vi "UI Controller.vi"(7 "Name (\"\" to Use UUID)":string="UI Controller") -> ()   [LabVIEW 2020]
uses:
  7d187395-4702-4f48-a3f4-ebc70eba639a.vi
  <userlib>/_NEVSTOP/Communicable State Machine(CSM)/AdvanceAPI/CSM - Revert Arguments-Safe String.vi
  <userlib>/_NEVSTOP/Communicable State Machine(CSM)/_Shared/Trim Single-line Text.vi
  <userlib>/_NEVSTOP/Communicable State Machine(CSM)/AdvanceAPI/CSM - Make String Arguments Safe.vi
  <userlib>/_NEVSTOP/Communicable State Machine(CSM)/AdvanceAPI/CSM - Break Down Multiple States String.vi
  <userlib>/_NEVSTOP/Communicable State Machine(CSM)/AdvanceAPI/CSM - Keywords.vi
  <userlib>/_NEVSTOP/Communicable State Machine(CSM)/addons/API-String-Arugments-Support/_Support/Data To API String Arguments.vi
  <userlib>/_NEVSTOP/Communicable State Machine(CSM)/Communicable State Machine.lvlib
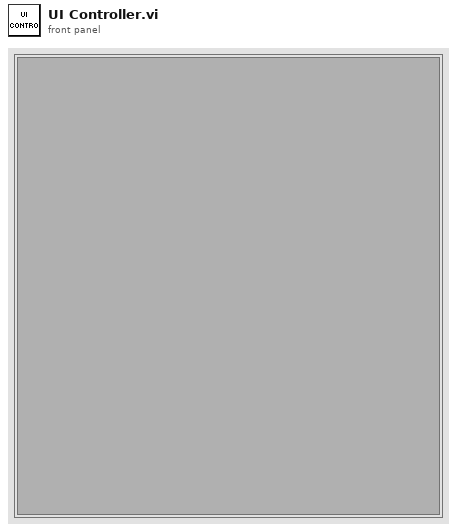
[diagram p1: front panel]
types:
  T1 = cluster{"Ref":cluster{"Name (\"\" to Use UUID)":refnum<vi>}, "Val":cluster{string}}
  T2 = cluster{"Current VI Reference":refnum<vi>, "Close Panel on Exit?":bool}
  T3 = cluster{"Core":cluster{"Current VI Reference":refnum<vi>, "Close Panel on Exit?":bool}, "1":cluster{"Ref":cluster{"Name (\"\" to Use UUID)":refnum<vi>}, "Val":cluster{string}}}
  T4 = enum32{"Invalid", "Standard", "Closed", "Hidden", "Minimized", "Maximized"}
  T5 = enum32{"invalid app kind", "Development System", "Run Time System", "Student Edition", "Embedded LabVIEW", "Evaluation", "Custom"}
  T6 = typedef "Communicable State Machine.lvlib/_CSM_Response Source Message.ctl" = cluster{"‘State":string, "’Arguments":string, "’Error":errorcluster}
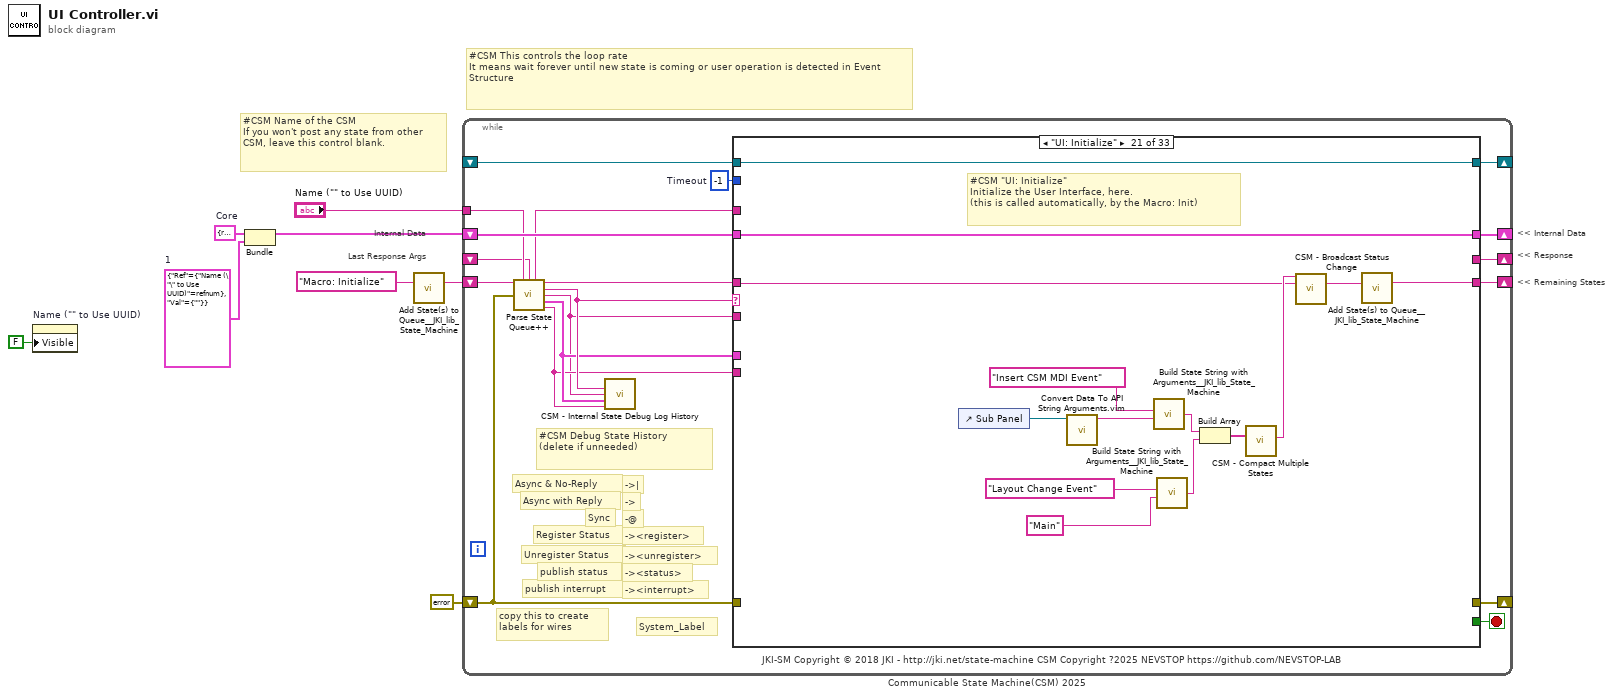
[diagram p0: block diagram]
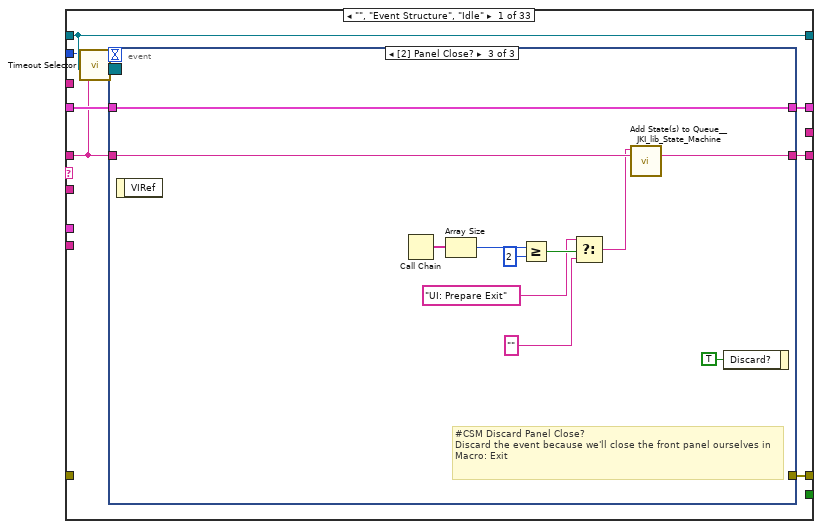
[diagram p2: hidden frame]
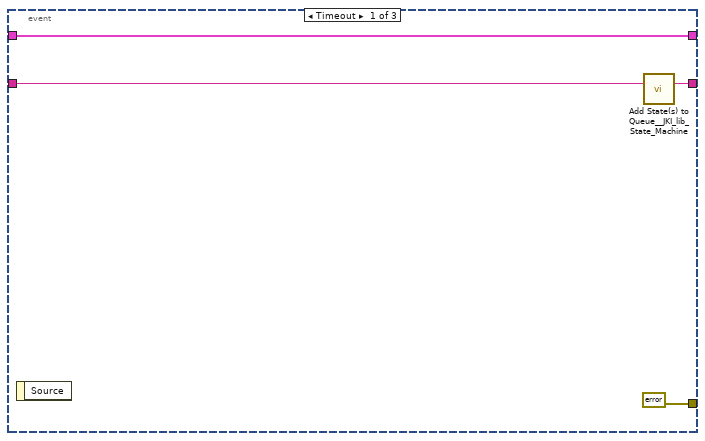
[diagram p3: hidden frame]
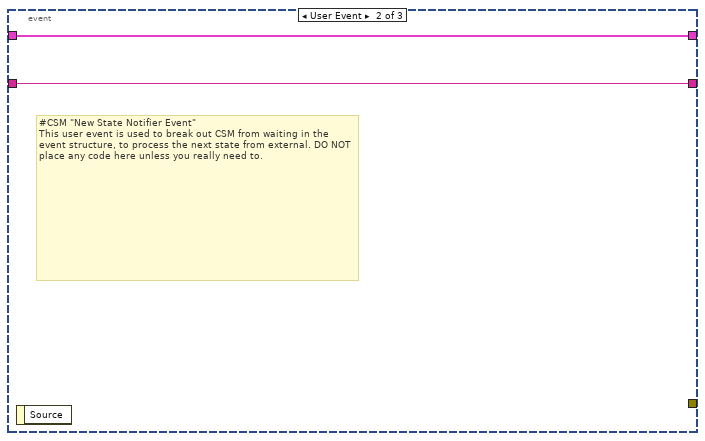
[diagram p4: hidden frame]
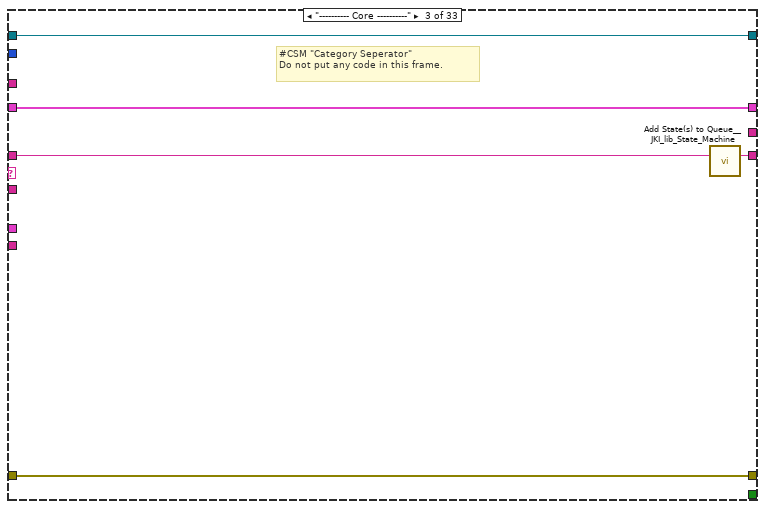
[diagram p6: hidden frame]
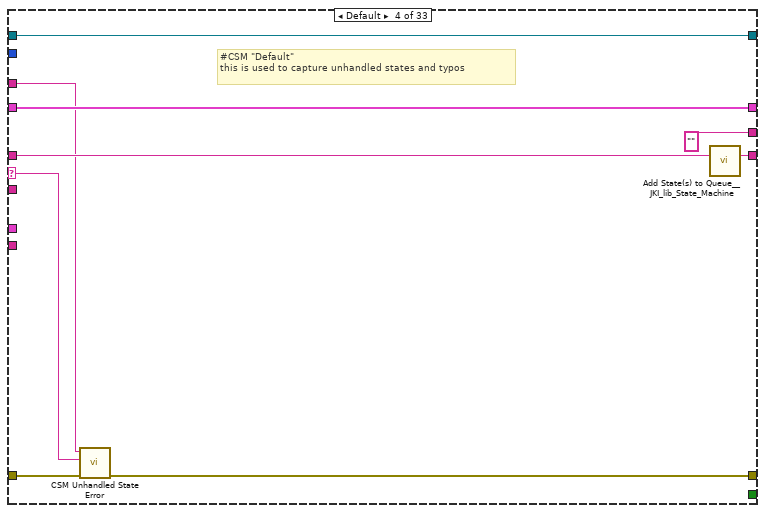
[diagram p7: hidden frame]
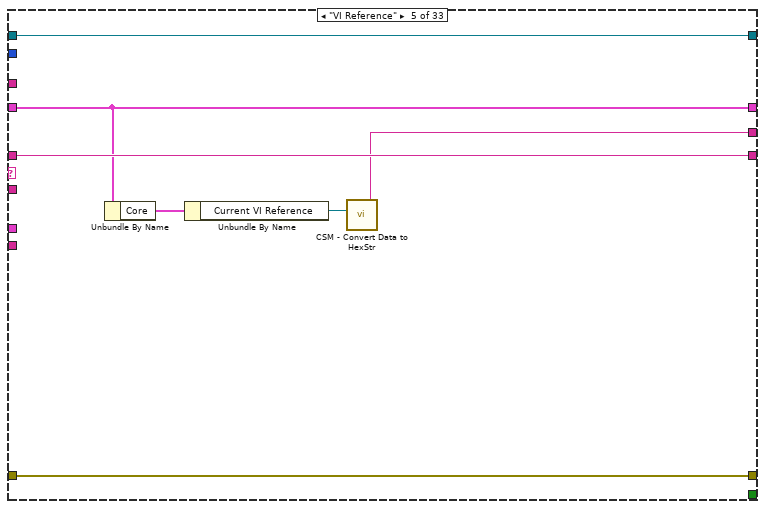
[diagram p8: hidden frame]
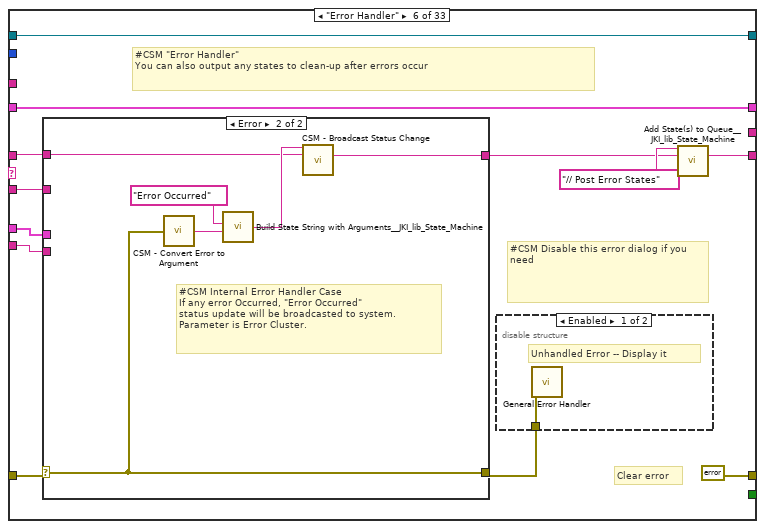
[diagram p9: hidden frame]
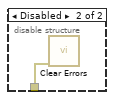
[diagram p10: hidden frame]
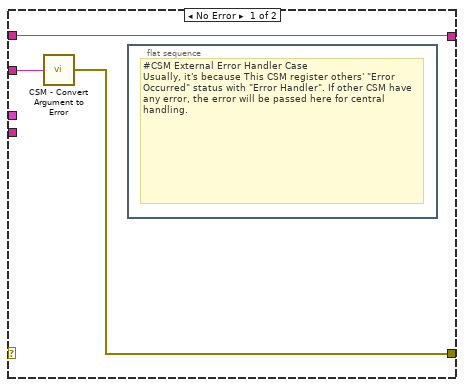
[diagram p11: hidden frame]
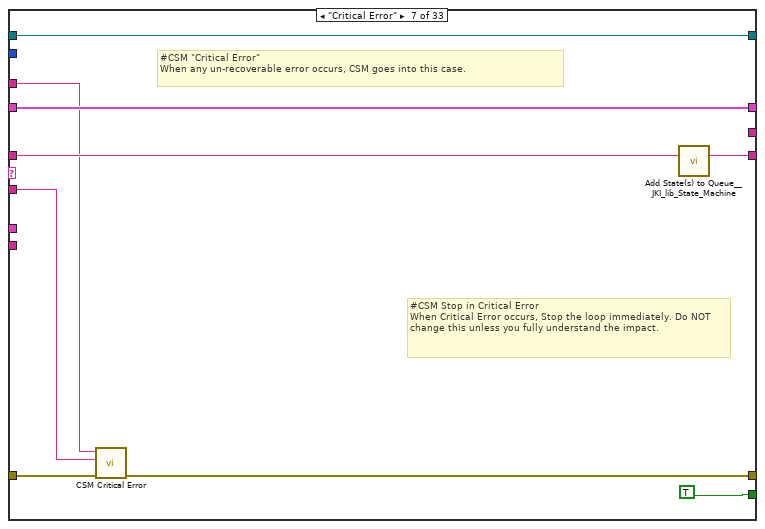
[diagram p12: hidden frame]
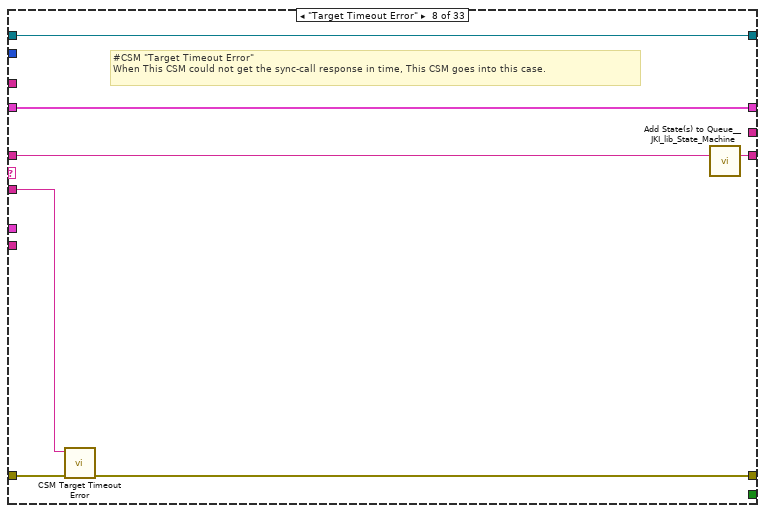
[diagram p13: hidden frame]
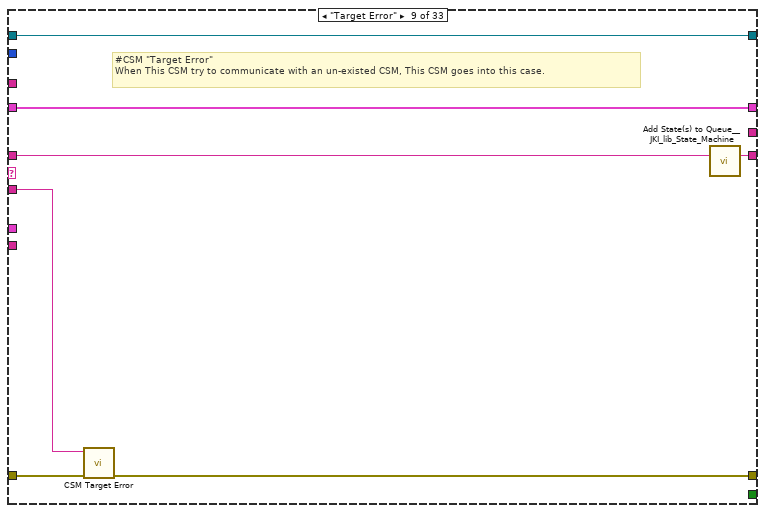
[diagram p14: hidden frame]
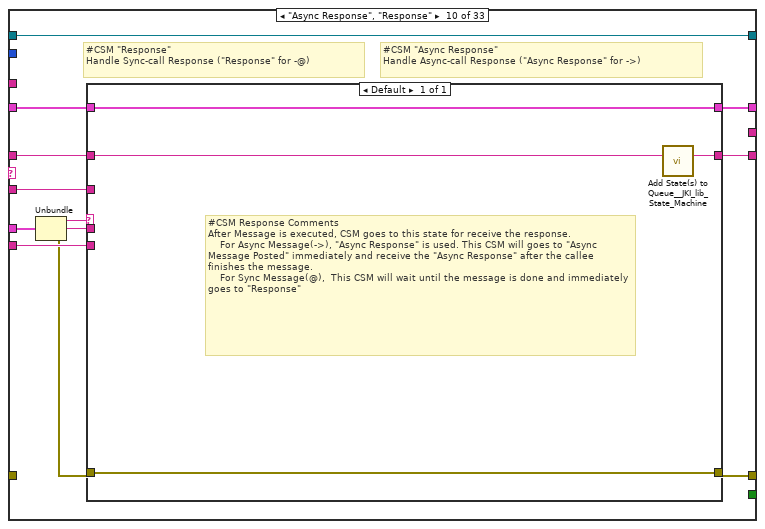
[diagram p15: hidden frame]
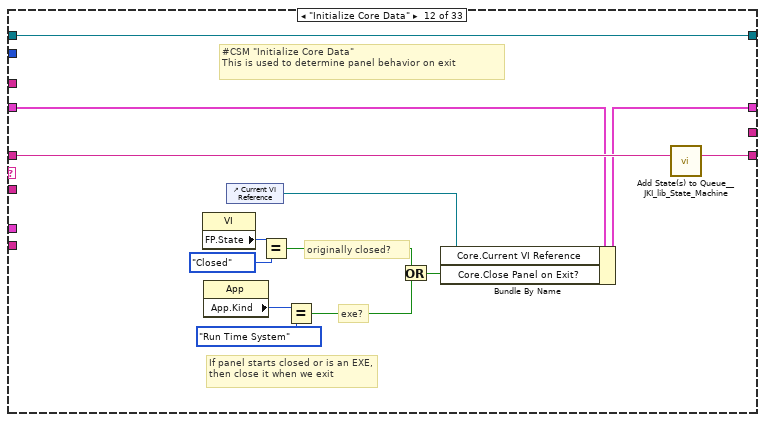
[diagram p17: hidden frame]
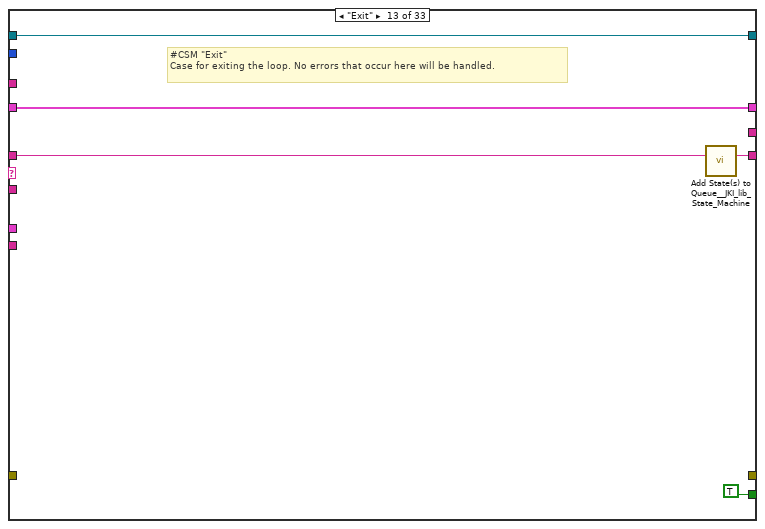
[diagram p18: hidden frame]
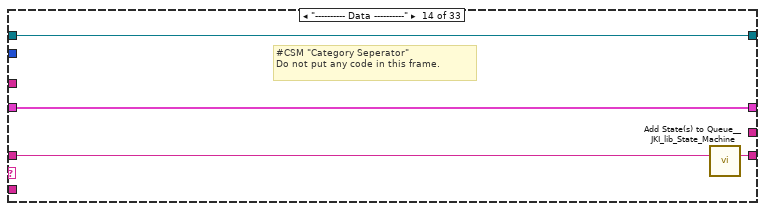
[diagram p19: hidden frame]
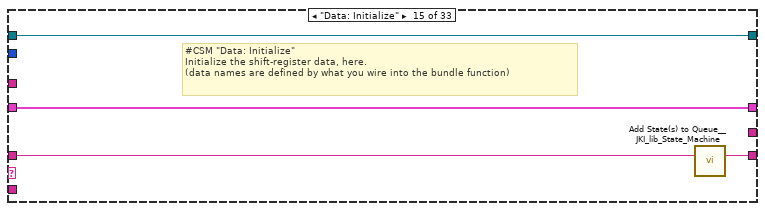
[diagram p20: hidden frame]
diagram:
  w7 = T1 {"Ref"={"Name (\"\" to Use UUID)"=refnum}, "Val"={""}}  # 1
  w6 = T2 {"Current VI Reference"=refnum, "Close Panel on Exit?"=FALSE}  # Core
  # "Last Response Args"
  # "Internal Data"
  # "<< Internal Data"
  # "<< Response"
  # "<< Remaining States"
  # "#CSM Name of the CSM\nIf you won't post any state from other CSM, leave this control blank."
  # "#CSM This controls the loop rate\nIt means wait forever until new state is coming or user operation is detected in Event Structure"
  n1 = property on="Name (\"\" to Use UUID)" class="Str"("Visible"=FALSE) -> ()  [unwired: 2 in, 2 out]
  n2 = Bundle("Core"=w6, "1"=w7) -> (w8:T3)  [unwired: 1 in]
  n3 = call <vilib>:"Add State(s) to Queue__JKI_lib_State_Machine.vi"("State(s) in (\"\")"="Macro: Initialize" ("Init State(\"Macro: Initialize\")")) -> ("States Out"=w2:string)  [unwired: 14 in]
  n4 = while "Communicable State Machine(CSM) 2025" {
    shift-right: [w22] -> _
    shift-left: w8 -> [w21]
    shift-right: [w25] -> _
    shift-left: errorcluster {"status"=FALSE, "code"=0, "source"=""} ("error out") -> [w19]
    shift-right: [w24] -> _
    shift-left: w2 -> [w26]
    tunnel: "Name (\"\" to Use UUID)" -> [w15]
    shift-right: [w18] -> _
    shift-left: _ -> [w10]
    shift-right: [w17] -> _
    shift-left: _ -> [w16]
    stop <- w23 stop-if-true
    w20 = -1  # Timeout
    # "#CSM Debug State History\n(delete if unneeded)"
    # "-><interrupt>"
    # "-><status>"
    # "-><unregister>"
    # "-><register>"
    # "-@"
    # "->"
    # "->|"
    # "publish interrupt"
    # "publish status"
    # "Unregister Status"
    # "Register Status"
    # "Sync"
    # "Async with Reply"
    # "Async & No-Reply"
    # "copy this to create labels for wires"
    # "System_Label"
    # "JKI-SM Copyright © 2018 JKI - http://jki.net/state-machine CSM Copyright ?2025 NEVSTOP https://github.com/NEVSTOP-LAB"
    n5 = call <userlib>:"Parse State Queue++.vi"("State Queue"=w26, "Name (\"\" to Use UUID)"=w15, "Response Arguments"=w10, "Previous Error"=w19) -> ("Name Used"=w11:string, "Remaining States"=w27:string, "Current State"=w14:string, "Arguments"=w9:string, "Additional Information"=w13:T6, "Source CSM"=w12:string)  [unwired: 6 in]
    n6 = call <userlib>:"CSM - Internal State Debug Log History.vi"("State"=w14, "Arguments (\"\")"=w9, ">> Response Source Message >>"=w13, "Source (\"\")"=w12) -> ()  [unwired: 11 in, 1 out]
    n7 = case shown="\"UI: Initialize\"" w14 {
      selector: w14 -> [_ _ _ w63 _ _ _ _ _ _ _ _ _ _ _ _ _ _ _ _ _ _ _ _ _ _ _ _ _ _ _ _ _]
      tunnel: w27 -> [w28 w55 w60 w69 w75 w81 w107 w115 w122 w132 w141 w154 w159 w163 w167 w173 w177 w184 w188 w192 w193 w208 w228 w239 w303 w304 w319 w322 w325 w330 w334 w338 w342]
      tunnel: w9 -> [_ _ _ _ _ w79 w103 w110 w118 w126 _ _ _ _ _ _ _ _ _ _ _ _ w224 w234 _ _ _ _ _ _ _ _ _]
      tunnel: w21 -> [w34 w54 w57 w67 w74 w87 w108 w113 w120 w130 w140 w148 w157 w161 w164 w169 w175 w183 w187 w190 w205 w215 w226 w236 w301 w307 w317 w321 w327 w329 w332 w336 w340]
      tunnel: [w33 _ w58 w61 w76 errorcluster {"status"=FALSE, "code"=0, "source"=""} ("error out") w100 w109 w116 w129 _ _ _ _ _ w170 _ w178 w186 _ _ _ w225 w237 _ _ _ _ _ _ _ _ _] -> w25
      tunnel: w19 -> [_ _ w58 w62 w76 w85 w101 w111 w117 _ _ _ _ _ _ _ _ _ _ _ _ _ _ _ _ _ _ _ _ _ _ _ _]
      tunnel: [w35 w55 w59 w68 w75 w83 w106 w114 w121 w133 w141 w153 w158 w162 w166 w172 w176 w184 w188 w191 w206 w209 w227 w238 w302 w308 w318 w322 w324 w330 w333 w337 w341] -> w24
      tunnel: [_ _ _ _ _ _ TRUE _ _ _ _ _ TRUE _ _ _ _ _ _ _ _ _ _ _ _ _ _ _ _ _ _ _ _] -> w23
      tunnel: [w32 w54 w57 w67 w74 w87 w108 w113 w120 w131 w140 w152 w157 w161 w164 w169 w175 w183 w187 w190 w205 w215 w226 w236 w301 w307 w317 w321 w327 w329 w332 w336 w340] -> w22
      tunnel: w20 -> [w30 _ _ _ _ _ _ _ _ _ _ _ _ _ _ _ _ _ _ _ _ _ _ _ _ _ _ _ _ _ _ _ _]
      tunnel: w12 -> [_ _ _ _ _ w78 _ _ _ w127 _ _ _ _ _ _ _ _ _ _ _ _ _ _ _ _ _ _ _ _ _ _ _]
      tunnel: w13 -> [_ _ _ _ _ w77 _ _ _ w128 _ _ _ _ _ _ _ _ _ _ _ _ _ _ _ _ _ _ _ _ _ _ _]
      tunnel: [_ _ _ "" w70 _ _ _ _ _ _ _ _ _ _ _ _ _ _ _ _ _ _ _ _ _ _ _ _ _ _ _ _] -> w18
      tunnel: [w31 w53 w56 w65 w73 w86 w104 w112 w119 w134 w139 w142 w155 w160 w165 w168 w174 w182 w185 w189 w204 w219 w223 w233 w300 w305 w311 w320 w326 w328 w331 w335 w339] -> w17
      tunnel: w16 -> [w31 w53 w56 w65 w73 w86 w104 w112 w119 w134 w139 w142 w155 w160 w165 w168 w174 _ w185 w189 w204 w219 w223 w233 w300 w305 w311 w320 w326 w328 w331 w335 w339]
      tunnel: w11 -> [_ _ _ w64 _ _ w102 _ _ _ _ _ _ _ _ _ _ w181 _ _ _ _ _ _ _ _ _ _ _ _ _ _ _]
      frame "", "Event Structure", "Idle" {
        n8 = call <userlib>:"Timeout Selector.vi"("Remaining States"=w28, "Timeout Expected"=w30) -> ("Timeout"=w29:i32)  [unwired: 5 in]
        n9 = event shown="[2] Panel Close?" {
          selector: w31 -> [_ _ _]
          dyn-events: _ -> [_ _ _]
          timeout: w29 -> [_ _ _]
          tunnel: w28 -> [w39 w40 w52]
          tunnel: [w38 w40 w51] -> w35
          tunnel: w34 -> [w37 w41 w50]
          tunnel: [errorcluster {"status"=FALSE, "code"=0, "source"=""} ("error out") _ _] -> w33
          tunnel: [w37 w41 w50] -> w32
          event Timeout {
            n10 = event-data() -> ()  [unwired: 1 in, 1 out]
            n11 = call <vilib>:"Add State(s) to Queue__JKI_lib_State_Machine.vi"("State(s) in (\"\")"=w39) -> ("States Out"=w38:string)  [unwired: 14 in]
          }
          event User Event {
            # "#CSM \"New State Notifier Event\"\nThis user event is used to break out CSM from waiting in the event structure, to process the next state from external. DO NOT place any code here unless you really need to."
            n12 = event-data() -> ()  [unwired: 1 in, 1 out]
          }
          event Panel Close? {
            # "#CSM Discard Panel Close?\nDiscard the event because we'll close the front panel ourselves in Macro: Exit"
            n13 = event-data() -> ()  [unwired: 1 in, 1 out]
            n14 = Call Chain() -> (call chain=w44:string[])
            n15 = Array Size(array=w44) -> (size(s)=w48:i32)
            n16 = Greater Or Equal?(x=w48, y=2) -> (x >= y?=w46:bool)
            n17 = Select(t="UI: Prepare Exit", s=w46, f="" ("t")) -> (s? t:f=w42:string)
            n18 = call <vilib>:"Add State(s) to Queue__JKI_lib_State_Machine.vi"("State(s) in Front (\"\")"=w42, "State(s) in (\"\")"=w52) -> ("States Out"=w51:string)  [unwired: 13 in]
            n19 = event-data("Discard?"=TRUE) -> ()  [unwired: 1 in, 1 out]
          }
        }
      }
      frame "CSM Documentation" {
        # "#CSM State Syntax\n\n// Comment line, all text to the right of “//” will be ignored\n// Local Message Example\nDoSth: DoA >> Arguments\n\n// Sync Call Example\nAPI: xxxx >> Arguments -@ TargetModule\n\n// Async Call Example\nAPI: xxxx >> Arguments -> TargetModule\n\n// Async Call without Reply Example\nAPI: xxxx >> Arguments ->| TargetModule\n\n// Broadcast normal status:\nStatus >> StatusArguments  -><status>\n\n// Broadcast Interrupt status:\nInterrupt >> StatusArguments  -><interrupt>\n\n// Register Source Module's status to Handler Module\nStatus@Source Module >> Handler Module@Handler Module -><register>\n\n// Unegister Source Module's status\nStatus@Source Module >> Handler Module -><unregister>"
        # "#CSM README FIRST\n\nCommunicable State Machine(CSM) is a LabVIEW application framework that builds upon JKI State Machine(JKISM). It follows the pattern of JKISM and extends the keywords to describe message communication between modules, including concepts such as Sync-Message, Async-Message, Subscription/Unsubscription of status - essential elements for creating reusable code modules. For more information, please visit the CSM wiki: https://nevstop-lab.github.io/CSM-Wiki/\n\nFor instructions on JKI State Machine, visit: \n    http://jki.net/state-machine/\nFor information about CSM, visit: \n    https://github.com/NEVSTOP-LAB"
        # "#CSM \"Documentation\"\nCase for holding CSM Documenation"
      }
      frame "---------- Core ----------" {
        # "#CSM \"Category Seperator\"\nDo not put any code in this frame."
        n20 = call <vilib>:"Add State(s) to Queue__JKI_lib_State_Machine.vi"("State(s) in (\"\")"=w60) -> ("States Out"=w59:string)  [unwired: 14 in]
      }
      frame Default {
        # "#CSM \"Default\"\nthis is used to capture unhandled states and typos"
        n21 = call <userlib>:"CSM Unhandled State Error.vi"("error in (no error)"=w62, "Undefined State"=w63, "CSM Name"=w64) -> ("error out"=w61:errorcluster)  [unwired: 8 in]
        n22 = call <vilib>:"Add State(s) to Queue__JKI_lib_State_Machine.vi"("State(s) in (\"\")"=w69) -> ("States Out"=w68:string)  [unwired: 14 in]
      }
      frame "VI Reference" {
        n23 = Unbundle By Name(w74) -> ("Core"=w72:T2)
        n24 = Unbundle By Name(w72) -> ("Current VI Reference"=w71:refnum<vi>)
        n25 = call <userlib>:"CSM - Convert Data to HexStr.vi"("Variant"=w71) -> ("HEX String (0-9,A-F)"=w70:string)  [unwired: 8 in]
      }
      frame "Error Handler" {
        # "#CSM Disable this error dialog if you need"
        # "#CSM \"Error Handler\"\nYou can also output any states to clean-up after errors occur"
        # "Clear error"
        n26 = case shown="Error" w85 {
          selector: w85 -> [_ w94]
          tunnel: [w92 w96] -> w82
          tunnel: w81 -> [w92 w95]
          tunnel: [w91 w94] -> w80
          tunnel: w79 -> [w93 _]
          tunnel: w78 -> [_ _]
          tunnel: w77 -> [_ _]
          frame No Error {
            n27 = call <userlib>:"CSM - Convert Argument to Error.vi"("Argument"=w93) -> ("Error"=w91:errorcluster)  [unwired: 4 in]
            n28 = flat-sequence {
              frame #0 {
                # "#CSM External Error Handler Case\nUsually, it's because This CSM register others' \"Error Occurred\" status with \"Error Handler\". If other CSM have any error, the error will be passed here for central handling."
              }
            }
          }
          frame Error {
            # "#CSM Internal Error Handler Case \nIf any error Occurred, \"Error Occurred\" \nstatus update will be broadcasted to system.\nParameter is Error Cluster."
            n29 = call <userlib>:"CSM - Convert Error to Argument.vi"("Error"=w94) -> ("Argument"=w98:string)  [unwired: 4 in]
            n30 = call <vilib>:"Build State String with Arguments__JKI_lib_State_Machine.vi"("Arguments (\"\")"=w98, "State"="Error Occurred" ("Status with Arguments")) -> ("State with Arguments"=w97:string)  [unwired: 4 in]
            n31 = call <userlib>:"CSM - Broadcast Status Change.vi"("Status With Arguments"=w97, "State Queue"=w95) -> ("Remaining States"=w96:string)  [unwired: 13 in]
          }
        }
        n32 = disable-structure shown="Enabled" {
          disable-tunnel: w80 -> [w89 w90]
          frame Enabled {
            # "Unhandled Error -- Display it"
            n33 = call <vilib>:"General Error Handler.vi"("error in (no error)"=w89) -> ()  [unwired: 10 in, 5 out]
          }
          frame Disabled {
            n34 = call <vilib>:"Clear Errors.vi"("error in (no error)"=w90) -> ()  [unwired: 5 in, 2 out]
          }
        }
        n35 = call <vilib>:"Add State(s) to Queue__JKI_lib_State_Machine.vi"("State(s) in Front (\"\")"="// Post Error States", "State(s) in (\"\")"=w82) -> ("States Out"=w83:string)  [unwired: 13 in]
      }
      frame "Critical Error" {
        # "#CSM \"Critical Error\"\nWhen any un-recoverable error occurs, CSM goes into this case."
        # "#CSM Stop in Critical Error\nWhen Critical Error occurs, Stop the loop immediately. Do NOT change this unless you fully understand the impact."
        n36 = call <userlib>:"CSM Critical Error.vi"("error in (no error)"=w101, "Arugments (As Reason)"=w103, "CSM Name"=w102) -> ("error out"=w100:errorcluster)  [unwired: 8 in]
        n37 = call <vilib>:"Add State(s) to Queue__JKI_lib_State_Machine.vi"("State(s) in (\"\")"=w107) -> ("States Out"=w106:string)  [unwired: 14 in]
      }
      frame "Target Timeout Error" {
        # "#CSM \"Target Timeout Error\"\nWhen This CSM could not get the sync-call response in time, This CSM goes into this case."
        n38 = call <userlib>:"CSM Target Timeout Error.vi"("error in (no error)"=w111, "Arguments (As CSM Name)"=w110) -> ("error out"=w109:errorcluster)  [unwired: 9 in]
        n39 = call <vilib>:"Add State(s) to Queue__JKI_lib_State_Machine.vi"("State(s) in (\"\")"=w115) -> ("States Out"=w114:string)  [unwired: 14 in]
      }
      frame "Target Error" {
        # "#CSM \"Target Error\"\nWhen This CSM try to communicate with an un-existed CSM, This CSM goes into this case."
        n40 = call <userlib>:"CSM Target Error.vi"("error in (no error)"=w117, "Arguments (As CSM Name)"=w118) -> ("error out"=w116:errorcluster)  [unwired: 9 in]
        n41 = call <vilib>:"Add State(s) to Queue__JKI_lib_State_Machine.vi"("State(s) in (\"\")"=w122) -> ("States Out"=w121:string)  [unwired: 14 in]
      }
      frame "Async Response", "Response" {
        # "#CSM \"Async Response\"\nHandle Async-call Response (\"Async Response\" for ->)"
        # "#CSM \"Response\"\nHandle Sync-call Response (\"Response\" for -@)"
        n42 = Unbundle(w128) -> ("‘State"=w125:string, "’Arguments"=w124:string, "’Error"=w123:errorcluster)
        n43 = case shown="Default" w125 {
          tunnel: [w135] -> w133
          tunnel: w132 -> [w136]
          tunnel: [w138] -> w131
          tunnel: w130 -> [w138]
          tunnel: [w137] -> w129
          tunnel: w123 -> [w137]
          tunnel: w127 -> [_]
          tunnel: w126 -> [_]
          tunnel: w124 -> [_]
          frame Default {
            # "#CSM Response Comments\nAfter Message is executed, CSM goes to this state for receive the response.\n    For Async Message(->), \"Async Response\" is used. This CSM will goes to \"Async Message Posted\" immediately and receive the \"Async Response\" after the callee finishes the message.\n    For Sync Message(@),  This CSM will wait until the message is done and immediately goes to \"Response\""
            n44 = call <vilib>:"Add State(s) to Queue__JKI_lib_State_Machine.vi"("State(s) in (\"\")"=w136) -> ("States Out"=w135:string)  [unwired: 14 in]
          }
        }
      }
      frame "Async Message Posted" {
        # "#CSM \"Async Message Posted\"\nAfter Async Message is posted (-> or ->| ), CSM goes to this state for post-action.\nYou can use Argument - State to tell which Async Message is called."
      }
      frame "Initialize Core Data" {
        # "#CSM \"Initialize Core Data\"\nThis is used to determine panel behavior on exit"
        # "originally closed?"
        # "exe?"
        # "If panel starts closed or is an EXE, then close it when we exit"
        n45 = property class="VI"() -> ("FP.State"=w145:T4)  [unwired: 2 in, 2 out]
        n46 = property class="App"() -> ("App.Kind"=w151:T5)  [unwired: 2 in, 2 out]
        n47 = control-ref of="Current VI Reference"() -> (w146:refnum<vi>)
        n48 = Equal?(x=w145, y=T4."Closed" ("Front Panel Window:State")) -> (x = y?=w143:bool)
        n49 = Equal?(x=w151, y=T5."Run Time System" ("Application:Kind")) -> (x = y?=w149:bool)
        n50 = Or(x=w143, y=w149) -> (x .or. y?=w147:bool)
        n51 = Bundle By Name(cluster=w148, "Core.Current VI Reference"=w146, "Core.Close Panel on Exit?"=w147) -> (w152:T3)
        n52 = call <vilib>:"Add State(s) to Queue__JKI_lib_State_Machine.vi"("State(s) in (\"\")"=w154) -> ("States Out"=w153:string)  [unwired: 14 in]
      }
      frame "Exit" {
        # "#CSM \"Exit\"\nCase for exiting the loop. No errors that occur here will be handled."
        n53 = call <vilib>:"Add State(s) to Queue__JKI_lib_State_Machine.vi"("State(s) in (\"\")"=w159) -> ("States Out"=w158:string)  [unwired: 14 in]
      }
      frame "---------- Data ----------" {
        # "#CSM \"Category Seperator\"\nDo not put any code in this frame."
        n54 = call <vilib>:"Add State(s) to Queue__JKI_lib_State_Machine.vi"("State(s) in (\"\")"=w163) -> ("States Out"=w162:string)  [unwired: 14 in]
      }
      frame "Data: Initialize" {
        # "#CSM \"Data: Initialize\"\nInitialize the shift-register data, here.\n(data names are defined by what you wire into the bundle function)"
        n55 = call <vilib>:"Add State(s) to Queue__JKI_lib_State_Machine.vi"("State(s) in (\"\")"=w167) -> ("States Out"=w166:string)  [unwired: 14 in]
      }
      frame "Data: Cleanup" {
        # "#CSM \"Data: Cleanup\"\nCleanup any data and references, here.\n(this is called automatically, by the Macro: Exit)"
        n56 = Unbundle By Name(w169) -> ("Core.Current VI Reference"=w171:refnum<vi>)
        n57 = Close Reference(reference=w171) -> (error out=w170:errorcluster)  [unwired: 1 in]
        n58 = call <vilib>:"Add State(s) to Queue__JKI_lib_State_Machine.vi"("State(s) in (\"\")"=w173) -> ("States Out"=w172:string)  [unwired: 14 in]
      }
      frame "---------- Events ----------" {
        # "#CSM \"Category Seperator\"\nDo not put any code in this frame."
        n59 = call <vilib>:"Add State(s) to Queue__JKI_lib_State_Machine.vi"("State(s) in (\"\")"=w177) -> ("States Out"=w176:string)  [unwired: 14 in]
      }
      frame "Events: Register" {
        # "#CSM \"Events: Register\"\nRegister user event. New Message Event is registered to break CSM waiting in event structure by default."
        # "#CSM Register New Message Event\nRegister message event to break Waiting in Event structure."
        n60 = call <userlib>:"CSM - Get New State Notifier Event.vi"("Name (\"\" to Use UUID)"=w181) -> ("error out"=w179:errorcluster, "New State Notifier Event"=w180:refnum<user-event>)  [unwired: 9 in]
        n61 = register-events(error in=w179, w180) -> (reference out=w182:refnum<event-registration>, error out=w178:errorcluster)  [unwired: 1 in]
      }
      frame "Events: Unregister" {
        # "#CSM \"Events: Unregister\"\nUnregister user event."
        n62 = Unregister For Events(event registration refnum=w185) -> (error out=w186:errorcluster)  [unwired: 1 in]
      }
      frame "---------- UI ----------" {
        # "#CSM \"Category Seperator\"\nDo not put any code in this frame."
        n63 = call <vilib>:"Add State(s) to Queue__JKI_lib_State_Machine.vi"("State(s) in (\"\")"=w192) -> ("States Out"=w191:string)  [unwired: 14 in]
      }
      frame "UI: Initialize" {
        # "#CSM \"UI: Initialize\"\nInitialize the User Interface, here.\n(this is called automatically, by the Macro: Init)"
        n64 = control-ref of="Sub Panel"() -> (w202:refnum<vi>)
        n65 = call "Convert Data To API String Arguments.vim"("Data"=w202) -> ("API String"=w203:string)  [unwired: 7 in, 1 out]
        n66 = call <vilib>:"Build State String with Arguments__JKI_lib_State_Machine.vi"("Arguments (\"\")"=w203, "State"="Insert CSM MDI Event") -> ("State with Arguments"=w197:string)  [unwired: 4 in]
        n67 = call <vilib>:"Build State String with Arguments__JKI_lib_State_Machine.vi"("Arguments (\"\")"="Main" ("y"), "State"="Layout Change Event") -> ("State with Arguments"=w196:string)  [unwired: 4 in]
        n68 = Build Array(w197, w196) -> (w195:string[])
        n69 = call <userlib>:"CSM - Compact Multiple States.vi"("Multiple States"=w195) -> ("States"=w194:string)  [unwired: 9 in]
        n70 = call <userlib>:"CSM - Broadcast Status Change.vi"("Status With Arguments"=w194, "State Queue"=w193) -> ("Remaining States"=w200:string)  [unwired: 13 in]
        n71 = call <vilib>:"Add State(s) to Queue__JKI_lib_State_Machine.vi"("State(s) in (\"\")"=w200) -> ("States Out"=w206:string)  [unwired: 14 in]
      }
      frame "UI: Prepare Exit" {
        w212 = "Main" ("y")
        n72 = Unbundle By Name(w215) -> ("Core.Current VI Reference"=w214:refnum<vi>)
        n73 = property class="VI"(reference=w214) -> ("Front Panel.Title"=w218:string)  [unwired: 1 in, 2 out]
        n74 = Not Equal?(x=w218, y=w212) -> (x != y?=w211:bool)
        n75 = case shown="True" w211 {
          tunnel: [_ w221] -> w207
          tunnel: w212 -> [_ w220]
          frame False {
          }
          frame True {
            n76 = call <vilib>:"Build State String with Arguments__JKI_lib_State_Machine.vi"("Arguments (\"\")"=w220, "State"="Layout Change Event" ("Status With Arguments")) -> ("State with Arguments"=w221:string)  [unwired: 4 in]
          }
        }
        n77 = Select(t="", s=w211, f="Macro: Exit") -> (s? t:f=w213:string)
        n78 = call <vilib>:"Add State(s) to Queue__JKI_lib_State_Machine.vi"("State(s) in Front (\"\")"=w213, "State(s) in (\"\")"=w208) -> ("States Out"=w210:string)  [unwired: 13 in]
        n79 = call <userlib>:"CSM - Broadcast Status Change.vi"("Status With Arguments"=w207, "State Queue"=w210) -> ("Remaining States"=w209:string)  [unwired: 13 in]
      }
      frame "UI: Cursor Set" {
        # "Argument"
        # "#CSM \"UI: Cursor Set\"\nSet and Unset Cursor Busy.\n(Usage: \"UI: Cursor Set >> Busy|Idle\")"
        n80 = disable-structure shown="TARGET_TYPE!=Windows" {
          disable-tunnel: [w230 _] -> w225
          disable-tunnel: w224 -> [w229 _]
          frame condition #0 (active) {
            n81 = case shown="\"Idle\", Default" w229 {
              tunnel: [w231 w232] -> w230
              frame "Idle", Default {
                n82 = call <vilib>:"Unset Busy.vi"() -> ("error out"=w231:errorcluster)  [unwired: 11 in]
              }
              frame "Busy" {
                n83 = call <vilib>:"Set Busy.vi"() -> ("error out"=w232:errorcluster)  [unwired: 10 in, 1 out]
              }
            }
          }
          frame condition #1 {
          }
        }
        n84 = call <vilib>:"Add State(s) to Queue__JKI_lib_State_Machine.vi"("State(s) in (\"\")"=w228) -> ("States Out"=w227:string)  [unwired: 14 in]
      }
      frame "UI: Front Panel State" {
        # "Argument"
        # "#CSM \"UI: Front Panel State\"\nSet Front Panel Open or Closed\n(Usage: \"UI: Front Panel State >> Open|Close\")"
        n85 = Unbundle By Name(w236) -> ("Core.Current VI Reference"=w235:refnum<vi>)
        n86 = case shown="\"Maximize\", \"Maximized\"" w234 {
          tunnel: [w246 w259 w270 w282 w294] -> w237
          tunnel: w235 -> [w245 w257 w269 w281 w293]
          frame "Open", "Standard", Default {
            w240 = T4."Standard" ("State")
            n87 = property class="VI"(reference=w245) -> (reference out=w243:refnum<vi>, error out=w244:errorcluster, "FP.State"=w242:T4)  [unwired: 1 in]
            n88 = Not Equal?(x=w242, y=w240) -> (x != y?=w241:bool)
            n89 = case shown="True" w241 {
              tunnel: [w250 w252] -> w246
              tunnel: w244 -> [w249 w252]
              tunnel: w243 -> [w248 _]
              tunnel: w240 -> [w247 _]
              frame True {
                n90 = invoke class="VI" method="FP.Open"(reference=w248, error in=w249, "Activate"=TRUE, "State"=w247) -> (error out=w250:errorcluster)  [unwired: 1 in, 4 out]
              }
              frame False {
              }
            }
          }
          frame "Close", "Closed" {
            n91 = property class="VI"(reference=w257) -> (reference out=w256:refnum<vi>, error out=w258:errorcluster, "FP.State"=w254:T4)  [unwired: 1 in]
            n92 = Not Equal?(x=w254, y=T4."Closed" ("Front Panel Window:State")) -> (x != y?=w253:bool)
            n93 = case shown="True" w253 {
              tunnel: [w260 w263] -> w259
              tunnel: w258 -> [w260 w262]
              tunnel: w256 -> [_ w261]
              frame False {
              }
              frame True {
                n94 = invoke class="VI" method="FP.Close"(reference=w261, error in=w262) -> (error out=w263:errorcluster)  [unwired: 1 in, 2 out]
              }
            }
          }
          frame "Hidden", "Hide" {
            w264 = T4."Hidden" ("State")
            n95 = property class="VI"(reference=w269) -> (reference out=w267:refnum<vi>, error out=w268:errorcluster, "FP.State"=w266:T4)  [unwired: 1 in]
            n96 = Not Equal?(x=w266, y=w264) -> (x != y?=w265:bool)
            n97 = case shown="True" w265 {
              tunnel: [w274 w275] -> w270
              tunnel: w268 -> [w273 w275]
              tunnel: w267 -> [w272 _]
              tunnel: w264 -> [w271 _]
              frame True {
                n98 = invoke class="VI" method="FP.Open"(reference=w272, error in=w273, "State"=w271) -> (error out=w274:errorcluster)  [unwired: 2 in, 4 out]
              }
              frame False {
              }
            }
          }
          frame "Minimize", "Minimized" {
            w276 = T4."Minimized" ("State")
            n99 = property class="VI"(reference=w281) -> (reference out=w279:refnum<vi>, error out=w280:errorcluster, "FP.State"=w278:T4)  [unwired: 1 in]
            n100 = Not Equal?(x=w278, y=w276) -> (x != y?=w277:bool)
            n101 = case shown="False" w277 {
              tunnel: [w286 w287] -> w282
              tunnel: w280 -> [w285 w287]
              tunnel: w279 -> [w284 _]
              tunnel: w276 -> [w283 _]
              frame True {
                n102 = invoke class="VI" method="FP.Open"(reference=w284, error in=w285, "State"=w283) -> (error out=w286:errorcluster)  [unwired: 2 in, 4 out]
              }
              frame False {
              }
            }
          }
          frame "Maximize", "Maximized" {
            w288 = T4."Maximized" ("State")
            n103 = property class="VI"(reference=w293) -> (reference out=w291:refnum<vi>, error out=w292:errorcluster, "FP.State"=w290:T4)  [unwired: 1 in]
            n104 = Not Equal?(x=w290, y=w288) -> (x != y?=w289:bool)
            n105 = case shown="True" w289 {
              tunnel: [w298 w299] -> w294
              tunnel: w292 -> [w297 w299]
              tunnel: w291 -> [w296 _]
              tunnel: w288 -> [w295 _]
              frame True {
                n106 = invoke class="VI" method="FP.Open"(reference=w296, error in=w297, "State"=w295) -> (error out=w298:errorcluster)  [unwired: 2 in, 4 out]
              }
              frame False {
              }
            }
          }
        }
        n107 = call <vilib>:"Add State(s) to Queue__JKI_lib_State_Machine.vi"("State(s) in (\"\")"=w239) -> ("States Out"=w238:string)  [unwired: 14 in]
      }
      frame "---------- Macro ----------" {
        # "#CSM \"Category Seperator\"\nDo not put any code in this frame."
        n108 = call <vilib>:"Add State(s) to Queue__JKI_lib_State_Machine.vi"("State(s) in (\"\")"=w303) -> ("States Out"=w302:string)  [unwired: 14 in]
      }
      frame "Macro: Initialize" {
        w306 = "Data: Initialize\nInitialize Core Data\nEvents: Register\nUI: Initialize\nUI: Front Panel State >> Open"  # Data: Initialize Initialize Core Data Events: Register UI: Initialize UI: Front Panel State >> Open
        # "#CSM \"Macro: Initialize\"\nInitialization Macro (This is called once, when the VI starts)"
        n109 = call <vilib>:"Add State(s) to Queue__JKI_lib_State_Machine.vi"("State(s) in Front (\"\")"=w306, "State(s) in (\"\")"=w304) -> ("States Out"=w308:string)  [unwired: 13 in]
      }
      frame "Macro: Exit" {
        # "#CSM \"Macro: Exit\"\nExit Macro (This is called once, when the VI exits)"
        n110 = Unbundle By Name(w317) -> ("Core.Close Panel on Exit?"=w316:bool)
        n111 = Select(t="UI: Front Panel State >> Close", s=w316, f="") -> (s? t:f=w313:string)
        n112 = call <vilib>:"Add State(s) to Queue__JKI_lib_State_Machine.vi"("State(s) in Front (\"\")"="//Exit Sub-Modules ", "State(s) in (\"\")"=w313, "State(s) at Back (\"\")"="Data: Cleanup\nEvents: Unregister\nExit") -> ("States Out"=w309:string)  [unwired: 12 in]
        n113 = call <vilib>:"Add State(s) to Queue__JKI_lib_State_Machine.vi"("State(s) in Front (\"\")"=w309, "State(s) in (\"\")"=w319) -> ("States Out"=w318:string)  [unwired: 13 in]
      }
      frame "---------- API ----------" {
        # "#CSM \"Category Seperator\"\nDo not put any code in this frame."
      }
      frame "API: Exit" {
        n114 = call <vilib>:"Add State(s) to Queue__JKI_lib_State_Machine.vi"("State(s) in Front (\"\")"="Macro: Exit" ("Remaining States"), "State(s) in (\"\")"=w325) -> ("States Out"=w324:string)  [unwired: 13 in]
      }
      frame "API: API2" {
      }
      frame "---------- Action ----------" {
        # "#CSM \"Category Seperator\"\nDo not put any code in this frame."
        n115 = call <vilib>:"Add State(s) to Queue__JKI_lib_State_Machine.vi"("State(s) in (\"\")"=w334) -> ("States Out"=w333:string)  [unwired: 14 in]
      }
      frame "Action: action1" {
        # "#CSM \"Internal State\"\nThis category is used for holding internal states"
        n116 = call <vilib>:"Add State(s) to Queue__JKI_lib_State_Machine.vi"("State(s) in (\"\")"=w338) -> ("States Out"=w337:string)  [unwired: 14 in]
      }
      frame "Action: action2" {
        # "#CSM \"Internal State\"\nThis category is used for holding internal states"
        n117 = call <vilib>:"Add State(s) to Queue__JKI_lib_State_Machine.vi"("State(s) in (\"\")"=w342) -> ("States Out"=w341:string)  [unwired: 14 in]
      }
    }
  }
